vi "Verify Arduino Libraries.vi"(8 "Error In":errorcluster, 10 "Arduino Base Path":path=path "C:/Program Files (x86)/Arduino") -> (0 "Error Out":errorcluster, 1 "Arduino IDE Found?":bool, 2 "Libraries Exst?":bool, 3 "Path to Arduino\\libraries":path)   [LabVIEW 2020, in "LMH-LINX.lvlib"]
uses:
  <vilib>/MakerHub/LINX/LMH-LINX.lvlib
  <vilib>/regexp/Match Regular Expression.xnode
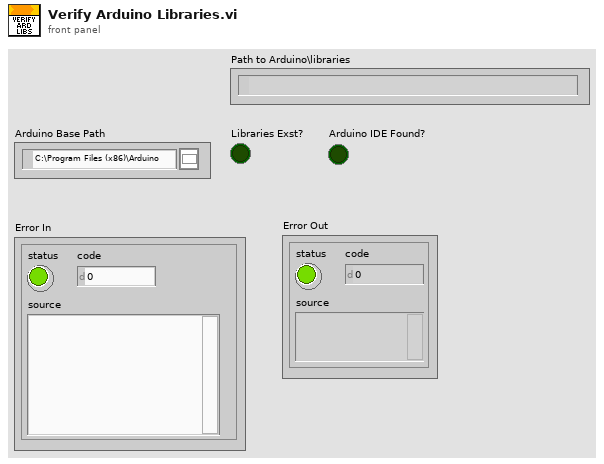
[diagram p1: front panel]
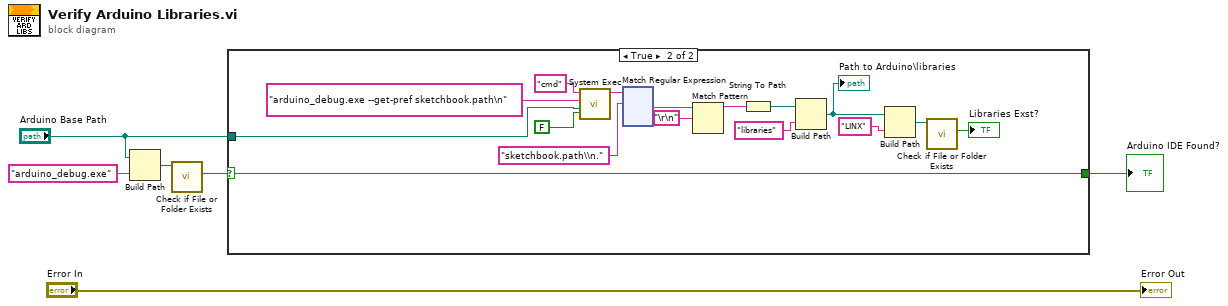
[diagram p0: block diagram]
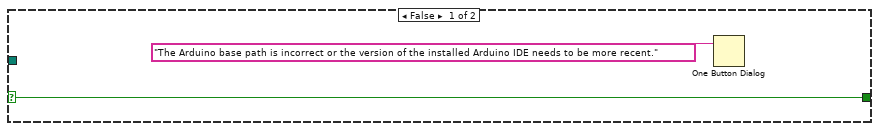
[diagram p2: hidden frame]
diagram:
  n1 = Build Path(base path="Arduino Base Path", name or relative path="arduino_debug.exe" ("command line")) -> (appended path=w2:path)
  n2 = call <vilib>:"Check if File or Folder Exists.vi"("path"=w2) -> ("file or folder exists?"=w5:bool)  [unwired: 8 in, 2 out]
  n3 = case shown="True" w5 {
    selector: w5 -> [w7 w9]
    tunnel: "Arduino Base Path" -> [_ w10]
    tunnel: [w7 w9] -> w1
    frame False {
      n4 = One Button Dialog(message="The Arduino base path is incorrect or the version of the installed Arduino IDE needs to be more recent.") -> ()  [unwired: 1 in, 1 out]
    }
    frame True {
      n5 = call <vilib>:"System Exec.vi"("run minimized? (F)"=FALSE, "working directory"=w10, "standard input"="arduino_debug.exe --get-pref sketchbook.path\n", "command line"="cmd") -> ("standard output"=w21:string)  [unwired: 4 in, 3 out]
      n6 = xnode "Match Regular Expression"("input string"=w21, "regular expression"="sketchbook.path\\n.") -> ("after match"=w13:string)  [unwired: 4 in, 4 out]
      n7 = Match Pattern(string=w13, regular expression="\r\n") -> (before substring=w11:string)  [unwired: 1 in, 3 out]
      n8 = String To Path(string=w11) -> (path=w19:path)
      n9 = Build Path(base path=w19, name or relative path="libraries") -> (appended path=w17:path)
      "Path to Arduino\\libraries" <- w17
      n10 = Build Path(base path=w17, name or relative path="LINX") -> (appended path=w15:path)
      n11 = call <vilib>:"Check if File or Folder Exists.vi"("path"=w15) -> ("file or folder exists?"=→"Libraries Exst?":bool)  [unwired: 8 in, 2 out]
    }
  }
  "Arduino IDE Found?" <- w1
  "Error Out" <- "Error In"
